vi "Shutdown HW.vi"(8 "error in (no error)":errorcluster, 11 "DAQmx Force Sensor in":refnum<class "DAQmx Force Sensor.lvclass">) -> (0 "error out":errorcluster, 3 "DAQmx Force Sensor out":refnum<class "DAQmx Force Sensor.lvclass">)   [LabVIEW 2020, in "DAQmx Force Sensor.lvclass"]
uses:
  DAQmx Force Sensor.lvclass
  DAQmx Force Sensor.lvclass/DAQmx Force Sensor.ctl
  Force Sensor.lvclass
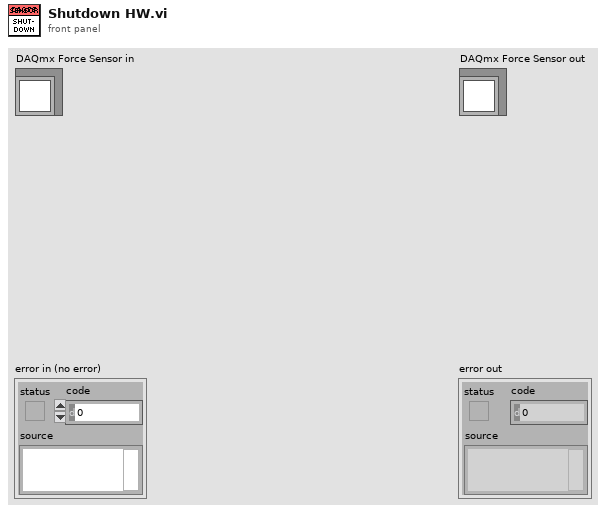
[diagram p1: front panel]
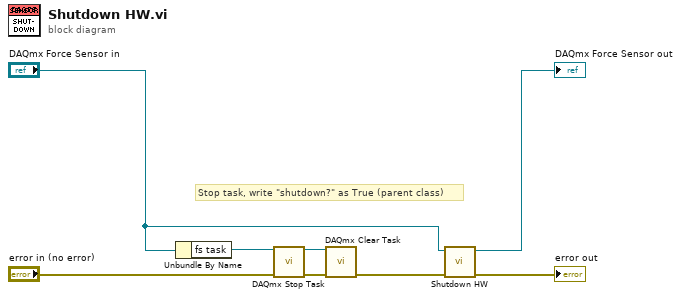
[diagram p0: block diagram]
diagram:
  # "Stop task, write \"shutdown?\" as True (parent class)"
  n1 = Unbundle By Name("DAQmx Force Sensor in") -> ("fs task"=w4:refnum<k21>)
  n2 = call <vilib>:"DAQmx Stop Task.vi"("task/channels in"=w4, "error in"="error in (no error)") -> ("task out"=w3:refnum<k21>, "error out"=w6:errorcluster)  [unwired: 12 in]
  n3 = call <vilib>:"DAQmx Clear Task.vi"("task in"=w3, "error in"=w6) -> ("error out"=w5:errorcluster)  [unwired: 13 in]
  n4 = call-parent "Shutdown HW.vi"("error in (no error)"=w5, "Force Sensor in"="DAQmx Force Sensor in") -> ("error out"=→"error out":errorcluster, "Force Sensor out"=→"DAQmx Force Sensor out":refnum<class "DAQmx Force Sensor.lvclass">)  [unwired: 8 in]
